vi "tm3samp_04_sequence_polling.vi"() -> ()   [LabVIEW 2011]
panel:
  out "Counter":i32
  out "Image":u16[][](graph)
  out "Frames Per Second":dbl
  in  "Quit":bool
  out "Error Out":errorcluster
  # "This is an example of how to check\nfor a new frame instead of waiting\nfor a new frame.  The counter will\nupdate while waiting for a new\nframe to arrive."
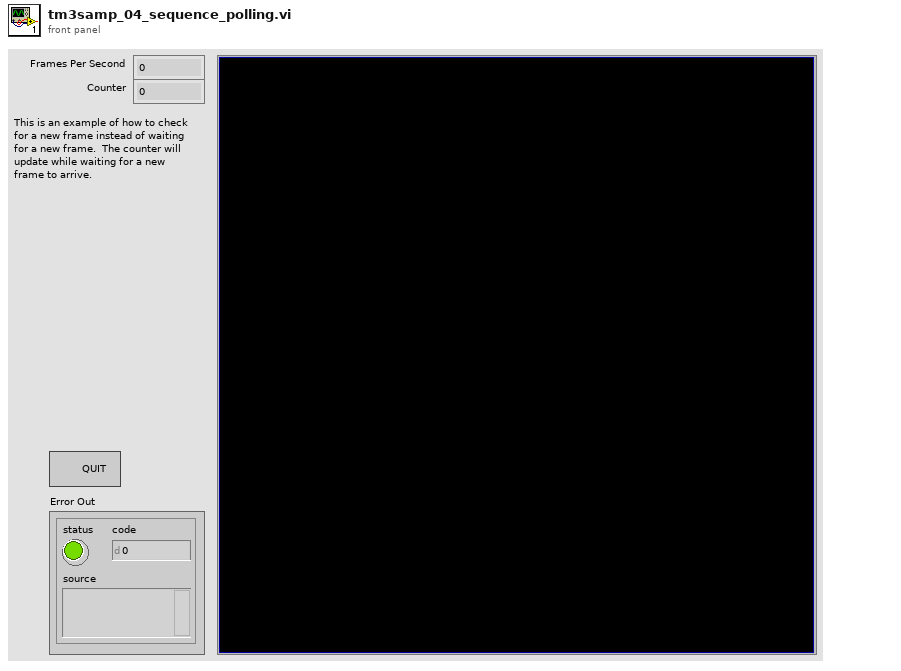
[diagram p1: front panel]
types:
  T1 = cluster{"height":u32, "width":u32, "datatype":u32}
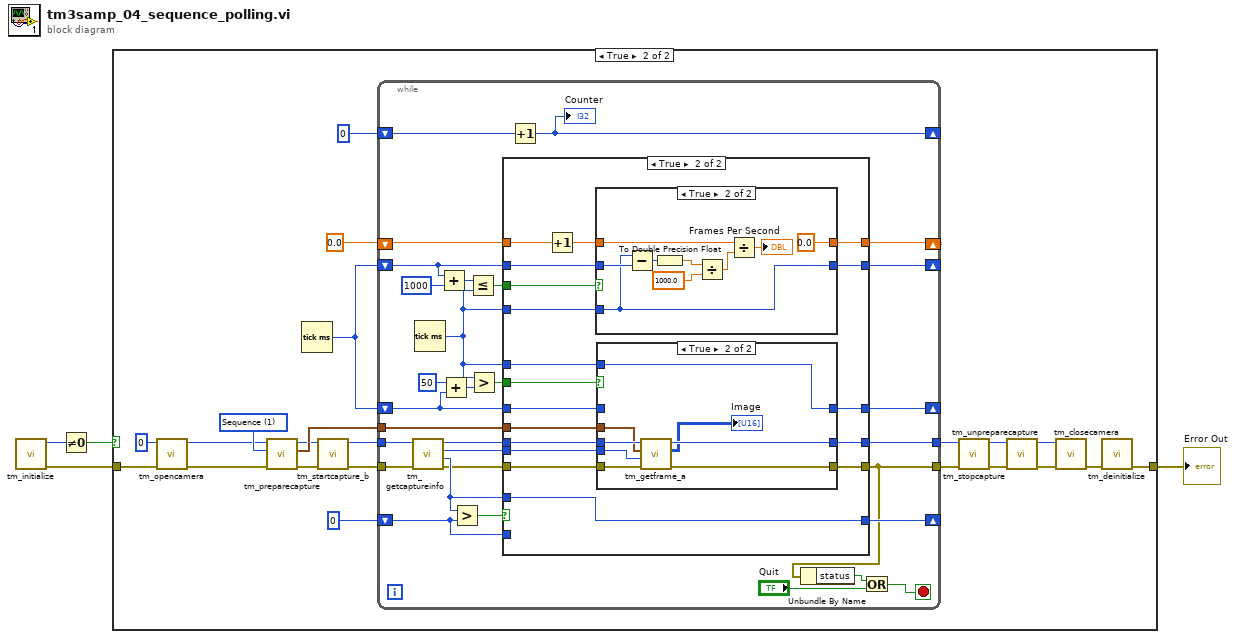
[diagram p0: block diagram]
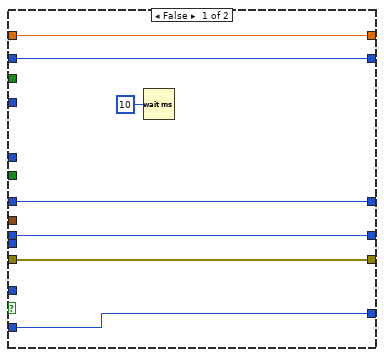
[diagram p3: hidden frame]
diagram:
  n1 = call <userlib>:"tm_initialize.vi"() -> ("error out"=w1:errorcluster, "Number Of Cameras"=w2:u32)  [unwired: 8 in, 2 out]
  n2 = Not Equal To 0?(x=w2) -> (x != 0?=w4:bool)
  n3 = case shown="True" w4 {
    tunnel: w1 -> [w5 w27]
    tunnel: [w5 w23] -> w3
    frame False {
    }
    frame True {
      w25 = 1 items=["Snap", "Sequence"] ("Capture mode")
      n4 = call <userlib>:"tm_opencamera.vi"("error in (no error)"=w27, "Camera Index"=u32 0) -> ("error out"=w6:errorcluster, "Handle out"=w7:u32)  [unwired: 7 in, 1 out]
      n5 = call <userlib>:"tm_preparecapture.vi"("error in (no error)"=w6, "Capture mode"=w25, "Handle in"=w7) -> ("error out"=w15:errorcluster, "Buffer Info"=w20:T1, "Handle out"=w14:u32)  [unwired: 5 in, 1 out]
      n6 = Tick Count (ms)() -> (millisecond timer value=w10:u32)
      n7 = call <userlib>:"tm_startcapture_b.vi"("error in (no error)"=w15, "Handle in"=w14) -> ("error out"=w12:errorcluster, "Handle out"=w13:u32)  [unwired: 8 in]
      n8 = while {
        tunnel: [w46] -> w18
        tunnel: [w45] -> w19
        tunnel: w20 -> [w44]
        tunnel: w13 -> [w53]
        tunnel: w12 -> [w52]
        shift-right: [w51] -> _
        shift-left: 0 -> [w50]
        shift-right: [w42] -> _
        shift-left: w10 -> [w30]
        shift-right: [w43] -> _
        shift-left: w10 -> [w31]
        shift-right: [w40] -> _
        shift-left: 0.0 -> [w41]
        shift-right: [w28] -> _
        shift-left: 0 -> [w29]
        stop <- w39 stop-if-true
        n9 = call <userlib>:"tm_getcaptureinfo.vi"("error in (no error)"=w52, "Handle in"=w53) -> ("error out"=w48:errorcluster, "Frame Count"=w54:i32, "Frame Index"=w47:i32, "Handle out"=w49:u32)  [unwired: 6 in]
        n10 = Tick Count (ms)() -> (millisecond timer value=w34:u32)
        n11 = Add(x=w30, y=u32 1000) -> (x+y=w35:u32)
        n12 = Add(x=u32 50, y=w31) -> (x+y=w38:u32)
        n13 = Greater?(x=w54, y=w50) -> (0:w55:bool)
        n14 = Less Or Equal?(x=w35, y=w34) -> (x <= y?=w32:bool)
        n15 = Greater?(x=w34, y=w38) -> (0:w33:bool)
        n16 = case shown="True" w55 {
          tunnel: w50 -> [w64 _]
          tunnel: [w64 w67] -> w51
          tunnel: w54 -> [_ w67]
          tunnel: w49 -> [w62 w82]
          tunnel: w48 -> [w63 w80]
          tunnel: w47 -> [_ w81]
          tunnel: [w63 w75] -> w45
          tunnel: [w62 w76] -> w46
          tunnel: w44 -> [_ w79]
          tunnel: w30 -> [w60 w78]
          tunnel: w31 -> [w61 w77]
          tunnel: [w61 w74] -> w43
          tunnel: [w60 w73] -> w42
          tunnel: w41 -> [w59 w65]
          tunnel: [w59 w72] -> w40
          tunnel: w34 -> [_ w71]
          tunnel: w34 -> [_ w70]
          tunnel: w33 -> [_ w69]
          tunnel: w32 -> [_ w68]
          frame False {
            n17 = Wait (ms)(milliseconds to wait=u32 10) -> ()  [unwired: 1 out]
          }
          frame True {
            n18 = Increment(x=w65) -> (x+1=w66:dbl)
            n19 = case shown="True" w68 {
              tunnel: w78 -> [w95 w98]
              tunnel: [w95 w96] -> w73
              tunnel: w66 -> [w94 w102]
              tunnel: w71 -> [_ w96]
              tunnel: [w94 0.0] -> w72
              frame False {
              }
              frame True {
                n20 = Subtract(x=w96, y=w98) -> (x-y=w97:u32)
                n21 = To Double Precision Float(number=w97) -> (double precision float=w104:dbl)
                n22 = Divide(x=w104, y=1000.0) -> (x/y=w101:dbl)
                n23 = Divide(x=w102, y=w101) -> (x/y=→"Frames Per Second":dbl)
              }
            }
            n24 = case shown="True" w69 {
              tunnel: w82 -> [w85 w93]
              tunnel: w80 -> [w84 w92]
              tunnel: w81 -> [_ w91]
              tunnel: w77 -> [w83 _]
              tunnel: w70 -> [_ w90]
              tunnel: [w85 w87] -> w76
              tunnel: [w84 w88] -> w75
              tunnel: [w83 w90] -> w74
              tunnel: w79 -> [_ w89]
              frame False {
              }
              frame True {
                n25 = call <userlib>:"tm_getframe_a.vi"("error in (no error)"=w92, "Frame Index"=w91, "Buffer Info"=w89, "Handle in"=w93) -> ("error out"=w88:errorcluster, "Data 16"=→"Image":u16[][], "Handle out"=w87:u32)  [unwired: 3 in, 2 out]
              }
            }
          }
        }
        n26 = Increment(x=w29) -> (x+1=w28:i32)
        "Counter" <- w28
        n27 = Unbundle By Name(w45) -> ("status"=w57:bool)
        n28 = Or(x=w57, y="Quit") -> (x .or. y?=w39:bool)
      }
      n29 = call <userlib>:"tm_stopcapture.vi"("error in (no error)"=w19, "Handle in"=w18) -> ("error out"=w16:errorcluster, "Handle out"=w17:u32)  [unwired: 8 in]
      n30 = call <userlib>:"tm_unpreparecapture.vi"("error in (no error)"=w16, "Handle in"=w17) -> ("error out"=w22:errorcluster, "Handle out"=w21:u32)  [unwired: 8 in]
      n31 = call <userlib>:"tm_closecamera.vi"("error in (no error)"=w22, "Handle in"=w21) -> ("error out"=w24:errorcluster)  [unwired: 9 in]
      n32 = call <userlib>:"tm_deinitialize.vi"("error in (no error)"=w24) -> ("error out"=w23:errorcluster)  [unwired: 10 in]
    }
  }
  "Error Out" <- w3
